vi "Sequence-StepStart.vi"(0 "MCListbox Refnum":refnum<vi>, 5 "Step Feedback":T1, 11 "error in (no error)":errorcluster) -> (4 "MCListbox Refnum(dup)":refnum<vi>, 15 "error out":errorcluster)   [LabVIEW 2020, in "CSMStand(Lite).lvlib"]
uses:
  CSMStand(Lite).lvlib
  <vilib>/Utility/miscctls.llb/LVRowAndColumnTypeDef.ctl
panel:
  # "Connector Pane"
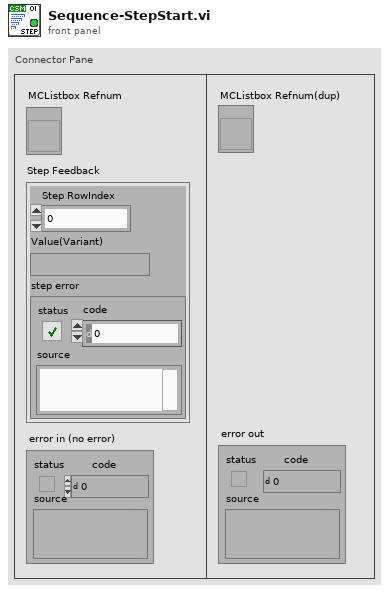
[diagram p1: front panel]
types:
  T1 = cluster{"Step RowIndex":i32, "Value(Variant)":variant, "step error":errorcluster}
  T2 = typedef "LVRowAndColumnTypeDef.ctl" = cluster{"Row":i32, "Column":i32}
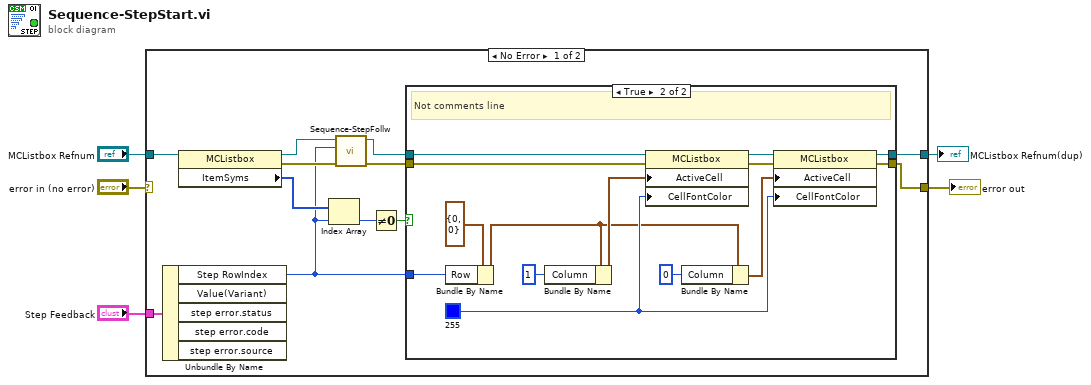
[diagram p0: block diagram]
diagram:
  n1 = case shown="No Error" "error in (no error)" {
    selector: "error in (no error)" -> [_ w35]
    tunnel: [w15 w35] -> w5
    tunnel: "MCListbox Refnum" -> [w17 w34]
    tunnel: [w16 w34] -> w2
    tunnel: "Step Feedback" -> [w11 _]
    frame No Error {
      n2 = Unbundle By Name(w11) -> ("Step RowIndex"=w6:i32)  [unwired: 4 out]
      n3 = property class="MCListbox"(reference=w17) -> (reference out=w8:refnum<vi>, error out=w10:errorcluster, "ItemSyms"=w14:i32[])  [unwired: 1 in]
      n4 = Index Array(array=w14, index=w6) -> (element=w13:i32)
      n5 = call "Sequence-StepFollw.vi"("error in (no error)"=w10, "Row Index"=w6, "MCListbox Refnum"=w8) -> ("error out"=w9:errorcluster, "MCListbox Refnum(dup)"=w7:refnum<vi>)  [unwired: 7 in]
      n6 = Not Equal To 0?(x=w13) -> (x != 0?=w12:bool)
      n7 = case shown="True" w12 {
        tunnel: [w19 w31] -> w16
        tunnel: [w18 w28] -> w15
        tunnel: w7 -> [w19 w24]
        tunnel: w9 -> [w18 w25]
        tunnel: w6 -> [_ w21]
        frame False {
        }
        frame True {
          w23 = u32 255 ("Active Cell:Cell Font:Color")
          # "Not comments line"
          n8 = Bundle By Name(cluster=T2 {"Row"=0, "Column"=0} ("Active Cell:Active Cell"), "Row"=w21) -> (w20:T2)
          n9 = Bundle By Name(cluster=w20, "Column"=1) -> (w32:T2)
          n10 = property class="MCListbox"(reference=w24, error in=w25, "ActiveCell"=w32, "CellFontColor"=w23) -> (reference out=w30:refnum<vi>, error out=w29:errorcluster)
          n11 = Bundle By Name(cluster=w20, "Column"=0) -> (w26:T2)
          n12 = property class="MCListbox"(reference=w30, error in=w29, "ActiveCell"=w26, "CellFontColor"=w23) -> (reference out=w31:refnum<vi>, error out=w28:errorcluster)
        }
      }
    }
    frame Error {
    }
  }
  "error out" <- w5
  "MCListbox Refnum(dup)" <- w2
